vi "Refnum_Names.vi"() -> ()   [LabVIEW 2018]
panel:
  in  "Compressor":string="Compressor"
  in  "CoPilot_Controller":string="CoPilot Controller"
  in  "Pilot_Controller":string="Pilot Controller"
  in  "Drive_Execute_Notifier":string="Drive Execute Notifier"
  in  "Drive_Set_Notifier":string="Drive Set Notifier"
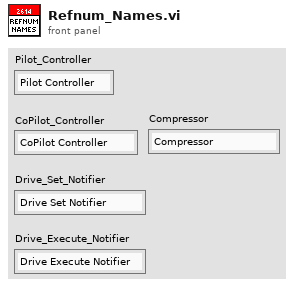
[diagram p1: front panel]
diagram:
